vi "AAL Resample (const to const, complex multi-channel).vi"(7 "reset?":bool, 8 "error in (no error)":errorcluster, 9 "config":T1={"new sample period"=0.0, "Timing Jitter"=enum."Interpolation", "first point location"=0.0, "prototype filter"={"h"=[], "Max Decimation"=1024}} {"prototype filter"."h" format="%.2f"; "first point location" format="%.2f"; "new sample period" format="%.2f"}, 10 "anti-aliasing?":bool=TRUE, 11 "X":cdb[][](array[numeric]) format="%.2f") -> (0 "error out":errorcluster, 2 "normalized t0":dbl, 3 "Y":cdb[][](array[numeric]) format="%.2f")   [LabVIEW 2017, in "NI_AALPro.lvlib"]
uses:
  <vilib>/Analysis/NI_AALPro.lvlib
  <resource>/lvanlys.dll
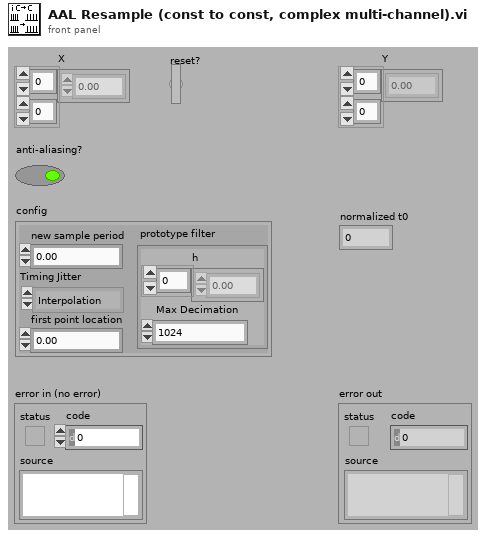
[diagram p1: front panel]
types:
  T1 = cluster{"new sample period":dbl, "Timing Jitter":enum32{"Interpolation", "Rounding"}, "first point location":dbl, "prototype filter":cluster{"h":dbl[], "Max Decimation":i32}}
  T2 = cluster{"precondition":cdb[], "preconditionLen":i32, "extractFilterBuffer":dbl[], "scaling":dbl, "extractFilterLeftLen":i32, "extractFilterRightLen":i32, "method":i32, "new sample period":dbl, "offset":dbl, "index":i32}
  T3 = cluster{"precondition":cdb[], "preconditionLen":i32, "extractFilterBuffer":dbl[], "scaling":dbl, "extractFilterLeftLen":i32, "extractFilterRightLen":i32, "method":i32, "new sample period":dbl, "offset":dbl, "index":i32}[]
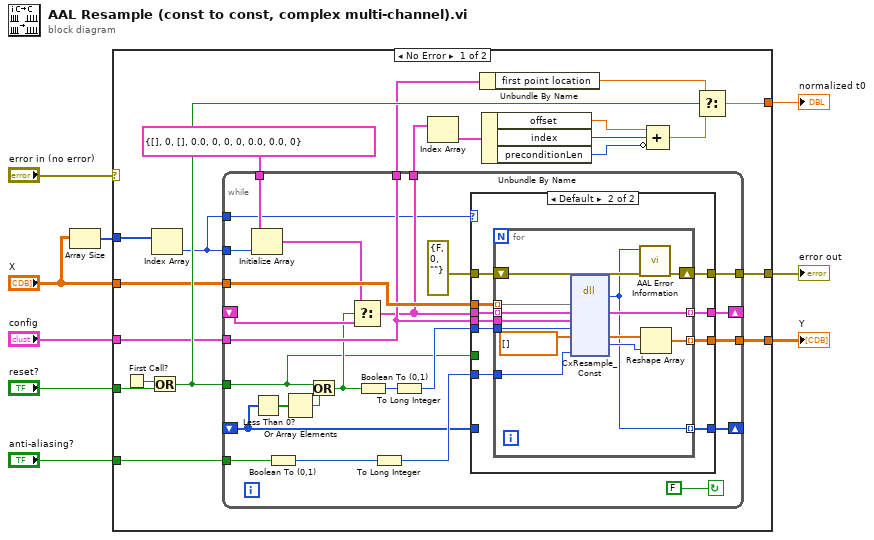
[diagram p0: block diagram]
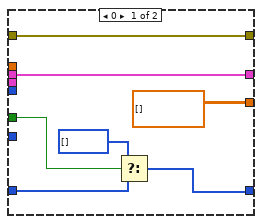
[diagram p2: hidden frame]
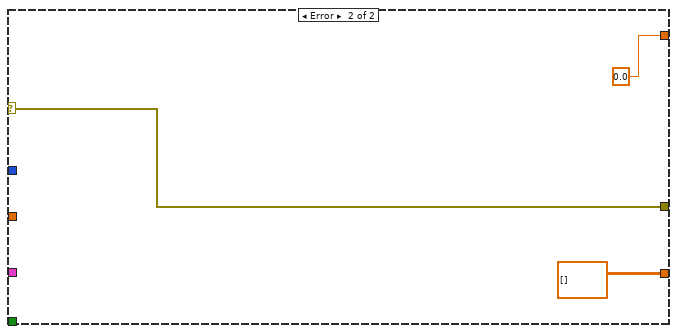
[diagram p3: hidden frame]
diagram:
  n1 = Array Size(array="X") -> (size(s)=w2:i32[])
  n2 = case shown="No Error" "error in (no error)" {
    selector: "error in (no error)" -> [_ w86]
    tunnel: "X" -> [w25 _]
    tunnel: "config" -> [w24 _]
    tunnel: "reset?" -> [w23 _]
    tunnel: [w22 0.0] -> w6
    tunnel: [w14 dbl[][] [] ("y")] -> w5
    tunnel: [w21 w86] -> w4
    tunnel: w2 -> [w13 _]
    tunnel: "anti-aliasing?" -> [w11 _]
    frame No Error {
      n3 = First Call?() -> (First Call?: T/F=w29:bool)
      n4 = Or(x=w29, y=w23) -> (x .or. y?=w28:bool)
      n5 = Index Array(array=w13) -> (element=w10:i32)  [unwired: 1 in]
      n6 = while {
        tunnel: w28 -> [w30]
        tunnel: w24 -> [w47]
        shift-left: _ -> [w51]
        shift-right: [w50] -> _
        tunnel: w25 -> [w52]
        tunnel: [w47] -> w27
        tunnel: [w43] -> w21
        tunnel: [w46] -> w16
        tunnel: [w45] -> w14
        tunnel: w10 -> [w42]
        tunnel: T2 {"precondition"=[], "preconditionLen"=0, "extractFilterBuffer"=[], "scaling"=0.0, "extractFilterLeftLen"=0, "extractFilterRightLen"=0, "method"=0, "new sample period"=0.0, "offset"=0.0, "index"=0} ("state") -> [w41]
        tunnel: w11 -> [w38]
        tunnel: w10 -> [w36]
        shift-right: [w35] -> _
        shift-left: _ -> [w31]
        stop <- FALSE continue-if-true
        n7 = Initialize Array(w41, w42) -> (w40:T3)
        n8 = Less Than 0?(x=w31) -> (x < 0?=w34:bool[])
        n9 = Boolean To (0,1)(Boolean=w38) -> (0, 1=w39:i16)
        n10 = Or Array Elements(Boolean array=w34) -> (logical OR=w33:bool)
        n11 = Or(x=w30, y=w33) -> (x .or. y?=w32:bool)
        n12 = Select(t=w40, s=w32, f=w51) -> (s? t:f=w46:T3)
        n13 = Boolean To (0,1)(Boolean=w32) -> (0, 1=w49:i16)
        n14 = To Long Integer(number=w39) -> (32bit integer=w37:i32)
        n15 = To Long Integer(number=w49) -> (32bit integer=w48:i32)
        n16 = case shown="Default" w36 {
          tunnel: w52 -> [_ w70]
          tunnel: [w59 w69] -> w50
          tunnel: w48 -> [_ w68]
          tunnel: w47 -> [_ w67]
          tunnel: w46 -> [w59 w66]
          tunnel: [cdb[][] [] ("y") w65] -> w45
          tunnel: errorcluster {"status"=FALSE, "code"=0, "source"=""} -> [w60 w64]
          tunnel: [w60 w63] -> w43
          tunnel: w37 -> [_ w62]
          tunnel: [w54 w61] -> w35
          tunnel: w31 -> [w56 _]
          tunnel: w30 -> [w57 _]
          frame 0 {
            n17 = Select(t=i32[] [], s=w57, f=w56) -> (s? t:f=w54:i32[])
          }
          frame Default {
            n18 = for {
              tunnel: w70 -> [w83] mode=indexing
              tunnel: [w81] -> w69 mode=indexing
              tunnel: w68 -> [w80]
              tunnel: w67 -> [w79]
              tunnel: w66 -> [w78] mode=indexing
              tunnel: [w75] -> w65 mode=indexing
              shift-right: [w73] -> w63
              shift-left: w64 -> [w74]
              tunnel: w62 -> [w72]
              tunnel: [w71] -> w61 mode=indexing
              n19 = dll-call lib="e:/builds/penguin/labview/branches/2017/dev/dist/resource/lvanlys.*" fn="CxResample_Const"("X"=w83, "state"=w78, "config"=w79, "reset"=w80, "y"=cdb[] [], "bandLimiting"=w72) -> (w71:i32, "state"=w81:T2, "y"=w77:cdb[], "out_len"=w76:i32)  [unwired: 8 in, 2 out]
              n20 = call <vilib>:"AAL Error Information.vi"("error in (no error)"=w74, "error code"=w71) -> ("error out"=w73:errorcluster)  [unwired: 9 in]
              n21 = Reshape Array(w77, w76) -> (w75:cdb[])
            }
          }
        }
      }
      n22 = Index Array(array=w16) -> (element=w15:T2)  [unwired: 1 in]
      n23 = Unbundle By Name(w27) -> ("first point location"=w26:dbl)
      n24 = Unbundle By Name(w15) -> ("offset"=w17:dbl, "index"=w20:i32, "preconditionLen"=w19:i32)
      n25 = Compound Arithmetic op=ADD(w17, w20, invert w19) -> (w18:dbl)
      n26 = Select(t=w26, s=w28, f=w18) -> (s? t:f=w22:dbl)
    }
    frame Error {
    }
  }
  "error out" <- w4
  "normalized t0" <- w6
  "Y" <- w5
